vi "Free.vi"(8 "No Error":errorcluster, 11 "Mem [void *]":i64 format="%.0x") -> (0 "Error Out":errorcluster)   [LabVIEW 2024, in "SDL3.lvlib" / "Stdinc.lvlib"]
doc: "<B>LabVIEW Implementation</B>\nThis function works event in case of error in.\n\n<B>Summary</B>\nFree allocated memory.\n\n<B>Remarks</B>\nThe pointer is no longer valid after this call and cannot be dereferenced anymore.\n\nIf mem is NULL, this function does nothing."
uses:
  Stdinc.lvlib
  Lib/SDL3-32.dll
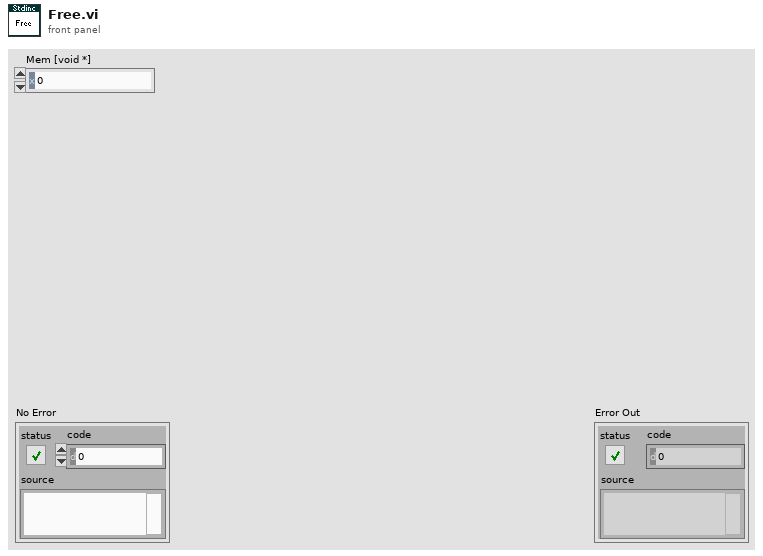
[diagram p1: front panel]
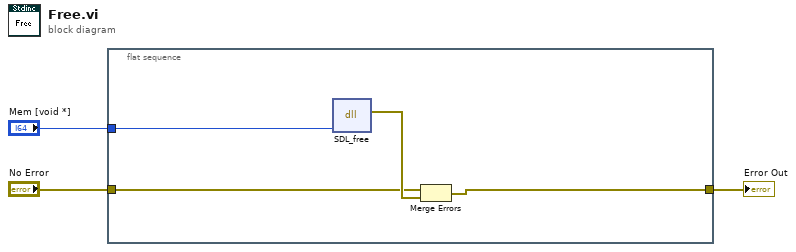
[diagram p0: block diagram]
diagram:
  n1 = flat-sequence {
    tunnel: "Mem [void *]" -> [w6]
    tunnel: [w5] -> w2
    tunnel: "No Error" -> [w4]
    frame #0 {
      n2 = dll-call lib="C:/Users/Thomas/Documents/Projects/LV-SDL3/Lib/SDL3-*.*" fn="SDL_free"("mem"=w6) -> (error out=w7:errorcluster)  [unwired: 5 in, 1 out]
      n3 = Merge Errors(w4, w7) -> (w5:errorcluster)
    }
  }
  "Error Out" <- w2
